vi "_getValueList.vi"   [LabVIEW 2022 SP3, in "openDAQ.lvlib" / "daqCoreTypes.lvlib" / "IDict.lvclass"]
uses:
  <instrlib>/openDAQ/Public/Classes/daqCoreTypes/IDict/IDict.lvclass
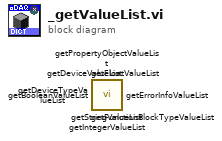
[diagram p0: block diagram]
diagram:
  n1 = call <instrlib>:"getStringValueList.vi"() -> ()  [unwired: 9 in, 3 out]
  n2 = call <instrlib>:"getFloatValueList.vi"() -> ()  [unwired: 9 in, 3 out]
  n3 = call <instrlib>:"getBooleanValueList.vi"() -> ()  [unwired: 9 in, 3 out]
  n4 = call <instrlib>:"getErrorInfoValueList.vi"() -> ()  [unwired: 9 in, 3 out]
  n5 = call <instrlib>:"getIntegerValueList.vi"() -> ()  [unwired: 9 in, 3 out]
  n6 = call <instrlib>:"getPropertyObjectValueList.vi"() -> ()  [unwired: 9 in, 3 out]
  n7 = call <instrlib>:"getDeviceValueList.vi"() -> ()  [unwired: 9 in, 3 out]
  n8 = call <instrlib>:"getFunctionBlockTypeValueList.vi"() -> ()  [unwired: 9 in, 3 out]
  n9 = call <instrlib>:"getDeviceTypeValueList.vi"() -> ()  [unwired: 9 in, 3 out]
